vi "tempconfigDO.vi"(1 "Temp Config in":cluster{"DO":refnum<k21>, "E_DO":errorcluster}, 2 "command":string) -> (0 "Temp Config out":cluster{"DO":refnum<k21>, "E_DO":errorcluster})   [LabVIEW 2015]
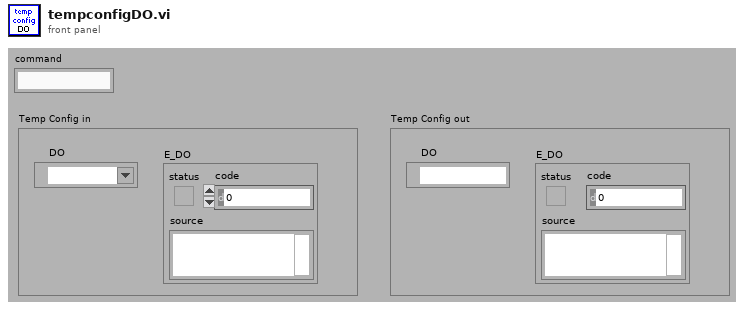
[diagram p1: front panel]
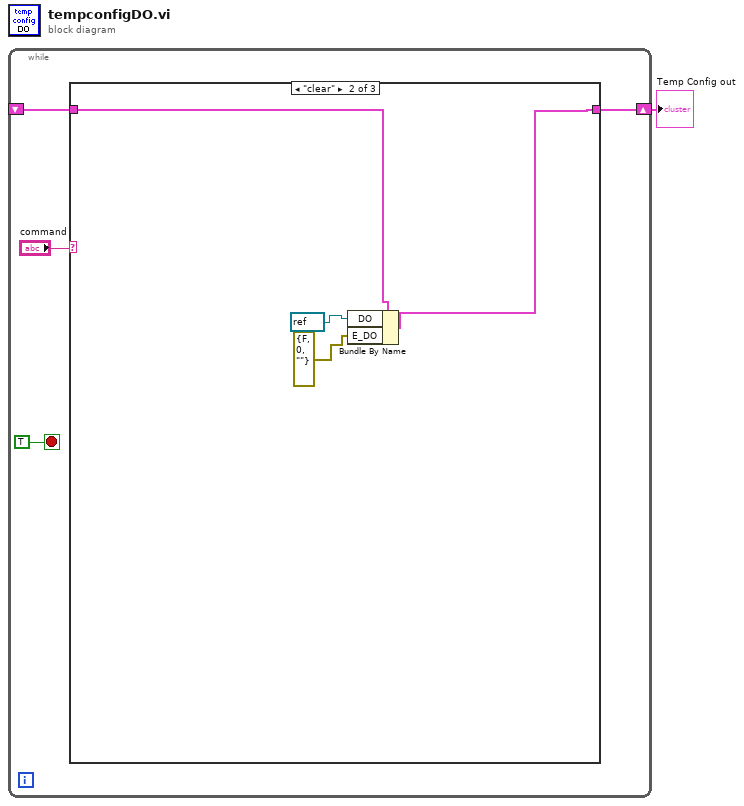
[diagram p0: block diagram]
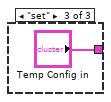
[diagram p3: hidden frame]
diagram:
  n1 = while {
    shift-right: [w3] -> w1
    shift-left: _ -> [w2]
    stop <- TRUE stop-if-true
    n2 = case shown="\"clear\"" "command" {
      tunnel: [w6 w10 "Temp Config in"] -> w3
      tunnel: w2 -> [w6 w9 _]
      frame "get", Default {
      }
      frame "clear" {
        n3 = Bundle By Name(cluster=w9, "DO"=refnum<k21> refnum ("XY"), "E_DO"=errorcluster {"status"=FALSE, "code"=0, "source"=""} ("E_AI")) -> (w10:cluster{"DO":refnum<k21>, "E_DO":errorcluster})
      }
      frame "set" {
      }
    }
  }
  "Temp Config out" <- w1
